vi "render_overlay_grid.vi"(6 "Grid Spacing":dbl, 7 "Image":T1) -> (3 "Image Out":T1)   [LabVIEW 2010]
uses:
  <vilib>/vision/Image Controls.llb/IMAQ Image.ctl
  red_tweezers_globals_INTERNAL.vi
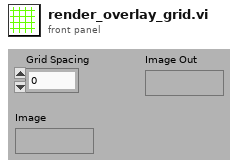
[diagram p1: front panel]
types:
  T1 = typedef "IMAQ Image.ctl" = refnum<image>
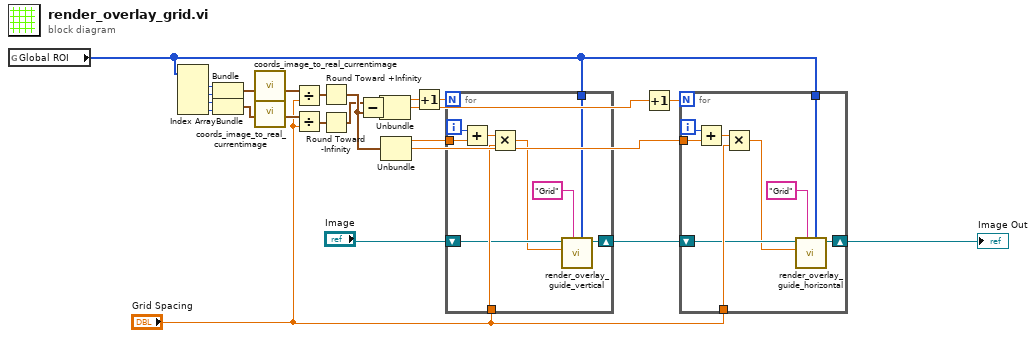
[diagram p0: block diagram]
diagram:
  n1 = global read "red_tweezers_globals_INTERNAL.vi" "Global ROI"() -> (w5:i32[])
  n2 = Index Array(array=w5) -> (element #1=w10:i32, element #2=w9:i32, element #3=w11:i32, element #4=w12:i32)  [unwired: 4 in]
  n3 = Bundle("Numeric"=w10, "Numeric"=w9) -> (w13:cluster{"Numeric":i32, "Numeric":i32})  [unwired: 1 in]
  n4 = Bundle("Numeric"=w11, "Numeric"=w12) -> (w14:cluster{"Numeric":i32, "Numeric":i32})  [unwired: 1 in]
  n5 = call "coords_image_to_real_currentimage.vi"("Position (pixels on image)"=w13) -> ("Position (real coords)"=w15:cluster{dbl, dbl, "Z":dbl})  [unwired: 9 in]
  n6 = call "coords_image_to_real_currentimage.vi"("Position (pixels on image)"=w14) -> ("Position (real coords)"=w16:cluster{dbl, dbl, "Z":dbl})  [unwired: 9 in]
  n7 = Divide(x=w15, y="Grid Spacing") -> (x/y=w17:cluster{dbl, dbl, "Z":dbl})
  n8 = Divide(x=w16, y="Grid Spacing") -> (x/y=w18:cluster{dbl, dbl, "Z":dbl})
  n9 = Round Toward +Infinity(x=w17) -> (ceil(x): smallest int >= x=w22:cluster{dbl, dbl, "Z":dbl})
  n10 = Round Toward -Infinity(1:w18) -> (0:w19:cluster{dbl, dbl, "Z":dbl})
  n11 = Subtract(x=w19, y=w22) -> (x-y=w21:cluster{dbl, dbl, "Z":dbl})
  n12 = Unbundle(w21) -> (w20:dbl, w1:dbl)  [unwired: 1 out]
  n13 = Unbundle(w22) -> (w23:dbl, w3:dbl)  [unwired: 1 out]
  n14 = Increment(x=w20) -> (x+1=w8:dbl)
  n15 = for {
    N: w8 -> [_]
    tunnel: w23 -> [w33]
    tunnel: "Grid Spacing" -> [w30]
    tunnel: w5 -> [w27]
    shift-right: [w28] -> w7
    shift-left: "Image" -> [w29]
    i -> [w32]
    n16 = Add(x=w32, y=w33) -> (x+y=w31:dbl)
    n17 = Multiply(x=w31, y=w30) -> (x*y=w25:dbl)
    n18 = call "render_overlay_guide_vertical.vi"("ROI"=w27, "Group"="Grid", "Position (real coords)"=w25, "Image"=w29) -> ("Image Out"=w28:T1)  [unwired: 5 in]
  }
  n19 = Increment(x=w1) -> (x+1=w2:dbl)
  n20 = for {
    N: w2 -> [_]
    tunnel: w3 -> [w42]
    tunnel: "Grid Spacing" -> [w39]
    tunnel: w5 -> [w35]
    shift-right: [w38] -> w6
    shift-left: w7 -> [w37]
    i -> [w41]
    n21 = Add(x=w41, y=w42) -> (x+y=w40:dbl)
    n22 = Multiply(x=w40, y=w39) -> (x*y=w34:dbl)
    n23 = call "render_overlay_guide_horizontal.vi"("ROI"=w35, "Group"="Grid", "Position (real coords)"=w34, "Image"=w37) -> ("Image Out"=w38:T1)  [unwired: 5 in]
  }
  "Image Out" <- w6
